vi "RB2 base station main demo 3.vi"() -> ()   [LabVIEW 2012]
panel:
  out "Num Posts":i32
  out "White dot\nLocation":T1(array[cluster])
  in  "File Path":path=path "C:/Users/GARLAND/Documents/Projects/Robotics II/Robotics 2 Spring 2014/Images with stations/photo 3.png"
  out "dot location string":string
  out "Dot Array":T2(array[cluster])
  out "All Found?":bool
  in  "stop":bool
  out "Mars image":T3(plugin-control)
  out "error out":errorcluster
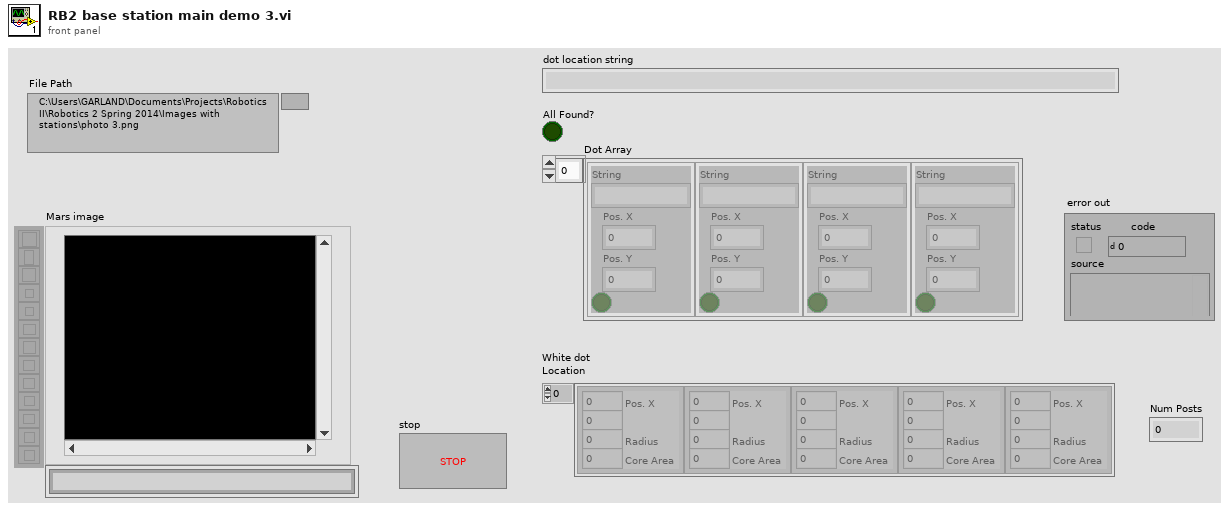
[diagram p1: front panel]
types:
  T1 = cluster{"Pos. X":i32, "Pos. Y":i32, "Radius":i32, "Core Area":i32}[]
  T2 = cluster{"String":string, "Pos. X":i32, "Pos. Y":i32, bool}[]
  T3 = typedef "IMAQ Image.ctl" = refnum<image>
  T4 = typedef "Image Type" = u32
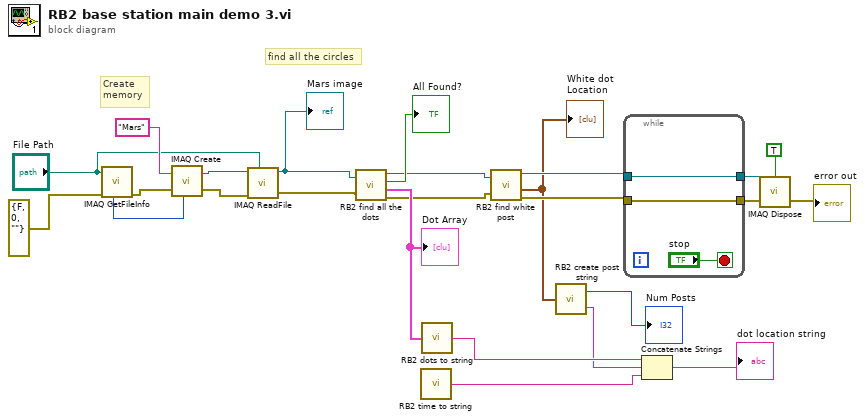
[diagram p0: block diagram]
diagram:
  # "find all the circles"
  # "Create \nmemory"
  n1 = call "IMAQ GetFileInfo"("error in (no error)"=errorcluster {"status"=FALSE, "code"=0, "source"=""}, "File Path"="File Path") -> ("error out"=w25:errorcluster, "Image Type"=w18:T4)  [unwired: 3 in, 5 out]
  n2 = call "IMAQ Create"("Image Name"="Mars", "Image Type"=w18, "error in (no error)"=w25) -> ("New Image"=w19:T3, "error out"=w22:errorcluster)  [unwired: 2 in]
  n3 = call "IMAQ ReadFile"("File Path"="File Path", "error in (no error)"=w22, "Image"=w19) -> ("error out"=w14:errorcluster, "Image Out"=w15:T3)  [unwired: 4 in, 3 out]
  "Mars image" <- w15
  n4 = call "RB2 find all the dots.vi"("Image In"=w15, "error in"=w14) -> ("Image Out"=w7:T3, "All Found?"=→"All Found?":bool, "Dot Array"=w12:T2, "error out"=w8:errorcluster)
  "Dot Array" <- w12
  n5 = call "RB2 time to string.vi"() -> ("time string"=w3:string)  [unwired: 1 in]
  n6 = call "RB2 dots to string.vi"("Dot Array"=w12) -> ("dot location string"=w11:string)
  n7 = call "RB2 find white post.vi"("Image In"=w7, "error in"=w8) -> ("Image Out"=w6:T3, "White dot\nLocation"=w4:T1, "error out"=w5:errorcluster)  [unwired: 1 out]
  "White dot\nLocation" <- w4
  n8 = call "RB2 create post string.vi"("White dot\nLocation"=w4) -> ("Num Posts"=→"Num Posts":i32, "Post String"=w2:string)
  n9 = while {
    tunnel: w6 -> [w27]
    tunnel: w5 -> [w26]
    tunnel: [w27] -> w17
    tunnel: [w26] -> w16
    stop <- "stop" stop-if-true
  }
  n10 = Concatenate Strings(w11, w2, w3) -> (→"dot location string":string)
  n11 = call "IMAQ Dispose"("All Images? (No)"=TRUE, "Image"=w17, "error in (no error)"=w16) -> ("error out"=→"error out":errorcluster)  [unwired: 3 in]
